vi "EyeTrackerFPGA (FPGA).vi"() -> ()   [LabVIEW 2012]
uses:
  <vilib>/Platform/TimedLoop/XDataNode/timing_clust.ctl
  <vilib>/Platform/TimedLoop/XDataNode/nitl_modes.ctl
  <vilib>/Platform/TimedLoop/XDataNode/wakeup.ctl
  Common/CL Configuration.ctl
  Common/CL Signal Mapping.ctl
  <vilib>/rvi/eio/common/nirviEmuTemplateMethod_errors.vi
  <vilib>/rvi/Emulation/niFpgaSctlEmulationRegisterWithScheduler.vi
  <vilib>/rvi/Emulation/niFpgaSctlEmulationScheduler.vi
  <vilib>/rvi/interface/RandomDataEmulation/nirviRandomDataFPGAFIFO.vi
  <vilib>/rvi/interface/RandomDataEmulation/niFpgaRandomDataHandleErrors.vi
  <vilib>/rvi/DataTransferAndStorage/Container/Common/niFpgaContainerGetUniqueNameForEmu.vi
  <vilib>/rvi/FIFO/Fifo_Resource/nirvififoEmulationSetSize.vi
  <vilib>/rvi/Emulation/niFpgaSctlEmulationFifoFullMgr.vi
  <vilib>/rvi/errors/niFpgaSetErrorForExecOnDevCompSimple.vi
  <vilib>/rvi/eio/common/nirviEmuReportErrorAndStop.vi
  Common/CL Data to Pixels/2 Tap 8-Bit.vi
  Common/CL Data to Pixels/2 Tap 10-Bit.vi
  <vilib>/rvi/Emulation/niFpgaSctlEmulationGlobalWrite.vi
  <vilib>/rvi/Emulation/niFpgaSctlEmulationResourceMgr.vi
  <vilib>/Platform/TimedLoop/XDataNode/XDataNode.xnode
  <vilib>/eio/EIONode/EIONode.xnode
  <vilib>/rvi/FXPMathLib/FxpInterpret/XNode/nifxpmath_Interpret.xnode
  <vilib>/rvi/DataTransferAndStorage/Container/XNode/niFpgaContainer.xnode
  <vilib>/rvi/interface/RandomDataEmulation/nirviRandomDataFpgaReadWriteTemplate.vi
  <vilib>/rvi/FIFO/Fifo_Resource/nirvififoEmulationRead.vi
  <vilib>/rvi/FIFO/Fifo_Resource/nirvififoEmulationWrite.vi
  <vilib>/Platform/TimedLoop/XDataNode/XDNodeRunTimeDep.lvlib
panel:
  in  "10-bit":bool
  out "Fixation.Fixated":bool
  in  "Fixation.MaxY":fxp<+/-,64,33> format="%.41g"
  in  "Fixation.MinY":fxp<+/-,64,33> format="%.41g"
  in  "Fixation.MaxX":fxp<+/-,64,33> format="%.41g"
  in  "Fixation.MinX":fxp<+/-,64,33> format="%.41g"
  in  "Fixation.MinimumEyeSize":u32
  out "AcqStatus.BufferToHostFull":bool
  out "AcqStatus.TenFrameTime":u32
  out "AcqStatus.DataAvailable":u32
  out "AcqStatus.PushedToHost":u32
  out "AcqStatus.PushedToMem":u32
  out "Acq Status.FrameWidth":u32
  out "Acq Status.FrameHeight":u32
  out "Acq Status.FrameNum":u32
  out "Acq Status.Acq'd Frame Width":u32
  out "Acq Status.Frames Acq'd":u32
  out "Acq Status.Acq'd Frame Height":u32
  out "Acq Status.DMA Write Timeout":bool
  out "Acq Status.Initialized":bool
  in  "EyePosition.Shift":i8=-2
  out "Timed Out?":bool
  out "Centroid.NumSent":i32
  out "Centroid.SumY":u32
  out "Centroid.SumX":u32
  out "Centroid.Size":u32
  out "Grabbed":bool
  out "Grabbing":bool
  in  "EyePosition.Color":u8=100
  in  "EyePosition.Send":bool
  in  "EyePosition.Threshold":u16=10
  out "TestX":u32
  out "TestY":u32
  in  "UART.Baud Rate":u8
  in  "UART.Transmit":bool
  in  "UART.Tx Data":u8[](array[numeric])=[0, 0, 0, 0, 0, 0, 0, 0, 0, 0] format="%02x"
  in  "UART.Set Baud Rate":bool
  in  "UART.Byte Mode":bool=TRUE
  out "UART.Rx Ready":bool
  out "UART.Break Indicator":bool
  out "UART.Framing Error":bool
  out "UART.Overrun Error":bool
  out "UART.Tx Ready":bool
  out "UART.Rx Data":u8 format="%02x"
  in  "UART.Receive":bool
  in  "Acq Control.Grab":bool
  in  "Acq Control.Acq":bool
  in  "Acq Control.IgnoreDVAL":bool
  in  "Acq Control.Clear Frame Cnt":bool
  in  "Acq Control.Initialize":bool
  in  "Trigger.Trigger Pulse Width (40 MHz Ticks)":u32=4000
  in  "Trigger.Send Software Trigger":bool
  in  "IO Module Config.CL DVAL Active High":bool=TRUE
  in  "IO Module Config.CL LVAL Active High":bool=TRUE
  in  "IO Module Config.CL FVAL Active High":bool=TRUE
  in  "IO Module Config.CL Spare Active High":bool=TRUE
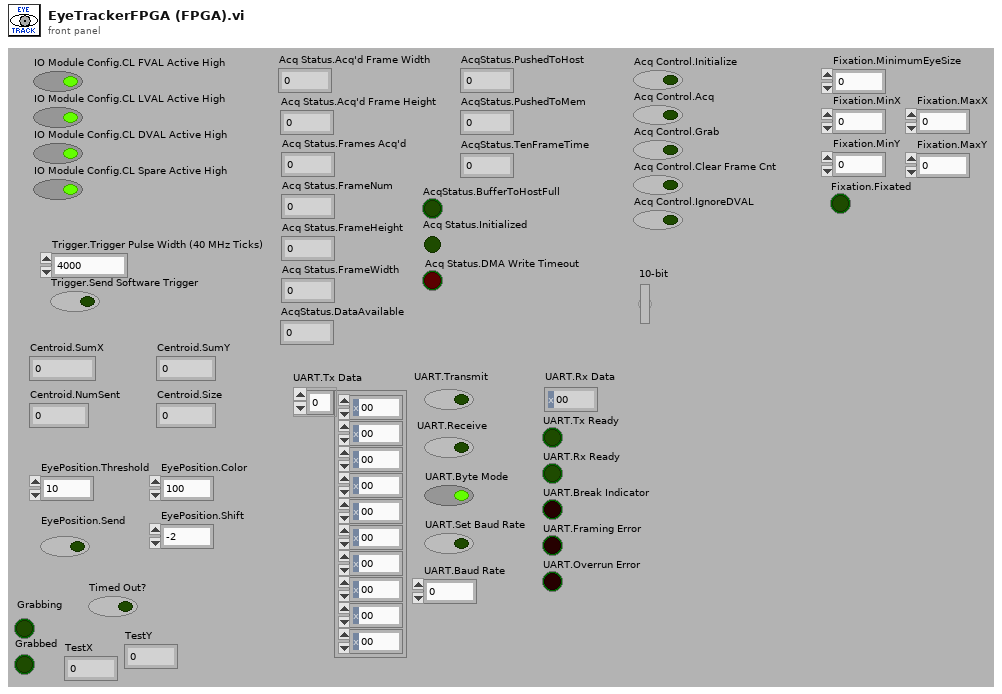
[diagram p1: front panel]
types:
  T1 = typedef "CL Signal Mapping.ctl" = enum8{"Standard", "Basler 10-tap", "Vosskühler 10-tap"}
  T2 = typedef "CL Configuration.ctl" = enum8{"Base", "Medium", "Full"}
  T3 = typedef "XDNodeRunTimeDep.lvlib/timing_clust.ctl" = cluster{"Expected End [f-1]":u64, "Actual End [f-1]":u64, "Finished Late? [f-1]":bool, "Expected End [i-1]":u64, "Actual End [i-1]":u64, "Finished Late? [i-1]":bool, "Expected Start [i]":u64, "Actual Start [i]":u64, "Expected Start [f]":u64, "Actual Start [f]":u64, "Source Name":string, "Structure Name":string, "Period":i64, "Deadline":i64, "Offset":i64, "Start":i64, "Priority":i32, "Timeout":i32, "Mode":T4, "Wakeup Reason":T5, "Error":errorcluster, "Source Type":string, "Secondary Source Type":string, "Global End Time":u64, "Global Start Time":u64, "Frame Duration":u64, "Iteration Duration":u64, "Assigned CPU":i32, "I/O Scan Engine Mode":u32}
  T4 = typedef "XDNodeRunTimeDep.lvlib/nitl_modes.ctl" = enum32{"No Change", "Process missed periods, maintain original phase", "Discard missed periods, maintain original phase", "Process missed periods, ignore original phase", "Discard missed periods, ignore original phase"}
  T5 = typedef "XDNodeRunTimeDep.lvlib/wakeup.ctl" = enum32{"Normal", "Aborted", "Asynchronous wakeup", "Timing source error", "Timed loop error", "Timeout"}
  T6 = enum16{"Idle", "WaitForPreviousEnd", "WaitForFrameRising", "WaitForFrameFalling", "CheckIfArmed"}
  T7 = cluster{"Tx Data":u8[], "Transmit":bool, "Receive":bool, "Byte Mode":bool, "Set Baud Rate":bool, "Baud Rate":u8}
  T8 = cluster{"Rx Data":u8, "Turn Off Transmit":bool, "Turn Off Receive":bool, "Turn Off Set Baud Rate":bool, "Tx Ready":bool, "Rx Ready":bool, "Break Indicator":bool, "Framing Error":bool, "Overrun Error":bool}
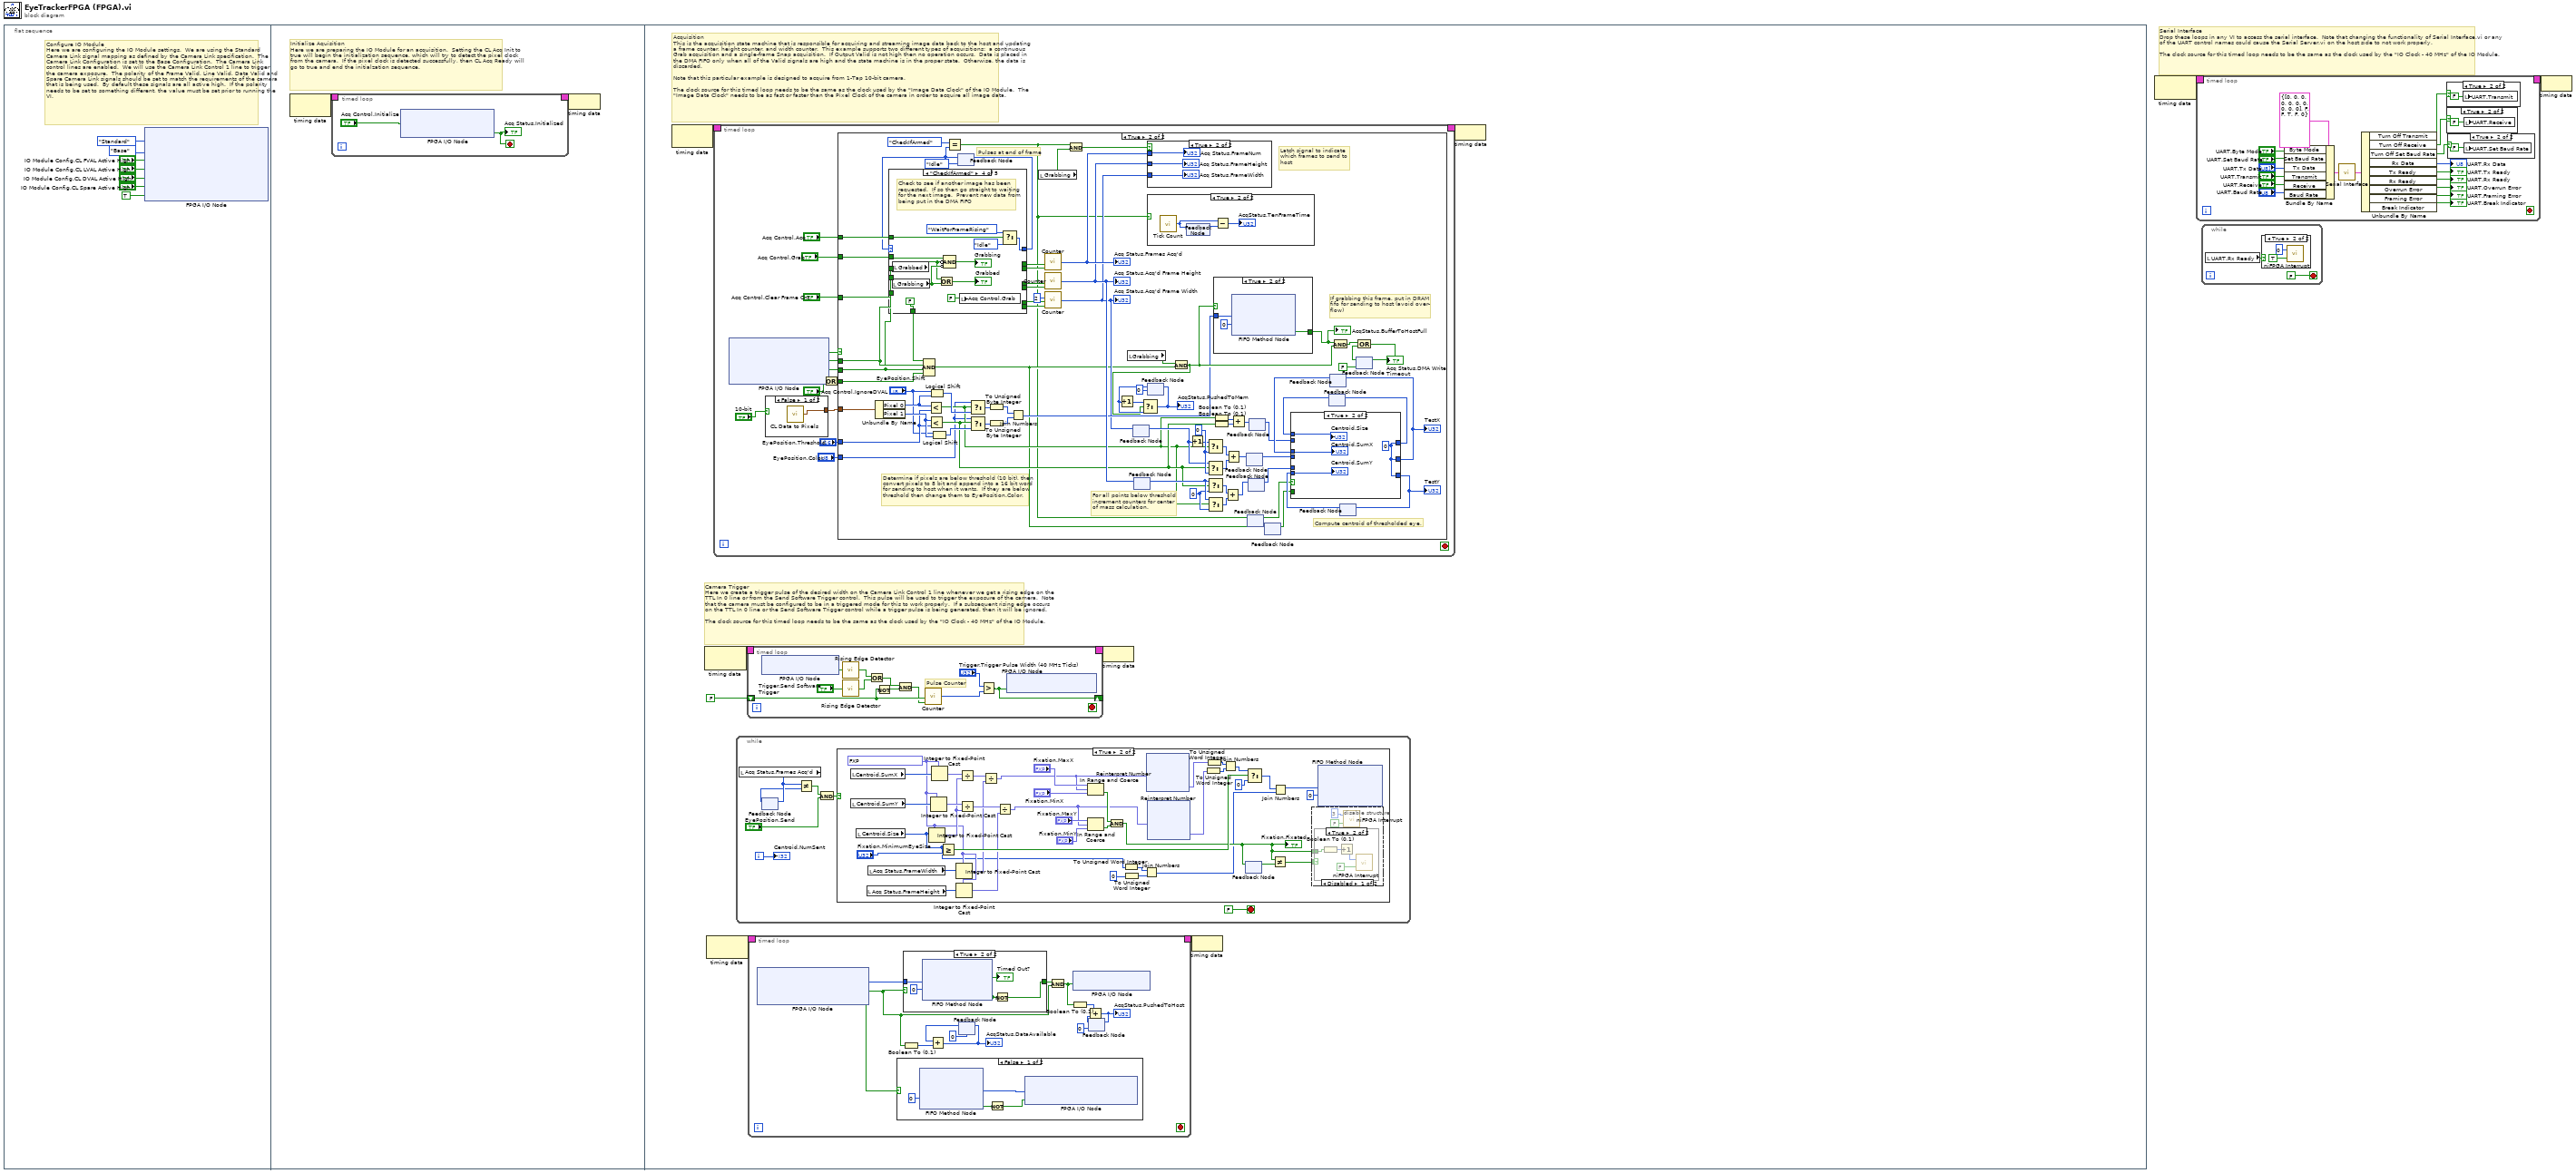
[diagram p0: block diagram]
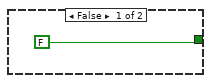
[diagram p7: hidden frame]
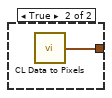
[diagram p11: hidden frame]
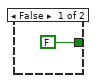
[diagram p14: hidden frame]
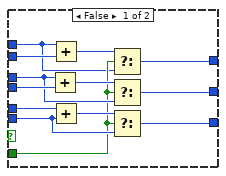
[diagram p16: hidden frame]
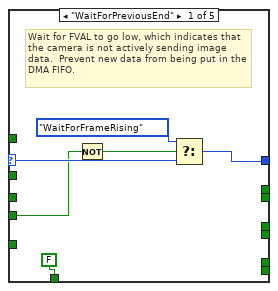
[diagram p17: hidden frame]
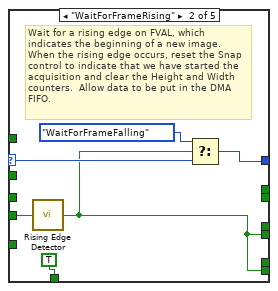
[diagram p18: hidden frame]
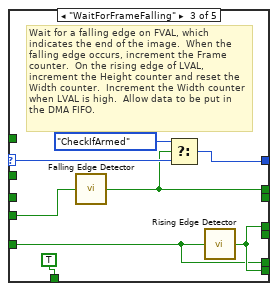
[diagram p19: hidden frame]
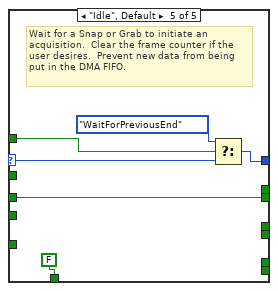
[diagram p20: hidden frame]
diagram:
  # "Serial Interface\nDrop these loops in any VI to access the serial interface.  Note that changing the functionality of Serial Interface.vi or any of the UART control names could cause the Serial Server.vi on the host side to not work properly.\n\nThe clock source for this timed loop needs to be the same as the clock used by the \"IO Clock - 40 MHz\" of the IO Module."
  n1 = flat-sequence {
    frame #0 {
      # "Configure IO Module\nHere we are configuring the IO Module settings.  We are using the Standard Camera Link signal mapping as defined by the Camera Link specification.  The Camera Link Configuration is set to the Base Configuration.  The Camera Link control lines are enabled.  We will use the Camera Link Control 1 line to trigger the camera exposure.  The polarity of the Frame Valid, Line Valid, Data Valid and Spare Camera Link signals should be set to match the requirements of the camera that is being used.  By default these signals are all active high.  If the polarity needs to be set to something different, the value must be set prior to running the VI."
      n2 = xnode "FPGA I/O Node"("IO Module\\CL Set Signal Mapping"=CL_Signal_Mapping."Standard" ("Camera Link Data Mapping"), "IO Module\\CL Set Configuration"=CL_Configuration."Base" ("CL Configuration"), "IO Module\\CL Set FVAL Active High"="IO Module Config.CL FVAL Active High", "IO Module\\CL Set LVAL Active High"="IO Module Config.CL LVAL Active High", "IO Module\\CL Set DVAL Active High"="IO Module Config.CL DVAL Active High", "IO Module\\CL Set Spare Active High"="IO Module Config.CL Spare Active High", "IO Module\\CL Control Enable"=TRUE ("IO Module\\CL Set Spare Active High")) -> ()  [unwired: 7 in, 7 out]
    }
    frame #1 {
      # "Initialize Aquisition\nHere we are preparing the IO Module for an acquisition.  Setting the CL Acq Init to true will begin the initialization sequence, which will try to detect the pixel clock from the camera.  If the pixel clock is detected successfully, then CL Acq Ready will go to true and end the initialzation sequence."
      n3 = node-c288() -> (w11:T3)  [unwired: 1 out]
      n4 = timed-loop {
        timing: w11 -> [_]
        timing-out: [_] -> w10
        stop <- w12 stop-if-true
        n5 = xnode "FPGA I/O Node"("IO Module\\CL Acq Init"="Acq Control.Initialize") -> ("IO Module\\CL Acq Ready"=w12:bool)  [unwired: 2 in, 2 out]
        "Acq Status.Initialized" <- w12
      }
      n6 = node-c288(w10) -> ()
    }
    frame #2 {
      # "Acquisition\nThis is the acquisition state machine that is responsible for acquiring and streaming image data back to the host and updating a frame counter, height counter, and width counter.  This example supports two different types of acquisitions:  a continuous Grab acquisition and a single-frame Snap acquisition.  If Output Valid is not high then no operation occurs.  Data is placed in the DMA FIFO only when all of the Valid signals are high and the state machine is in the proper state.  Otherwise, the data is discarded.\n\nNote that this particular example is designed to acquire from 1-Tap 10-bit camera.\n\nThe clock source for this timed loop needs to be the same as the clock used by the \"Image Data Clock\" of the IO Module.  The \"Image Data Clock\" needs to be as fast or faster than the Pixel Clock of the camera in order to acquire all image data."
      # "Camera Trigger\nHere we create a trigger pulse of the desired width on the Camera Link Control 1 line whenever we get a rising edge on the TTL In 0 line or from the Send Software Trigger control.  This pulse will be used to trigger the exposure of the camera.  Note that the camera must be configured to be in a triggered mode for this to work properly.  If a subsequent rising edge occurs on the TTL In 0 line or the Send Software Trigger control while a trigger pulse is being generated, then it will be ignored. \n\nThe clock source for this timed loop needs to be the same as the clock used by the \"IO Clock - 40 MHz\" of the IO Module."
      n7 = node-c288() -> (w24:T3)  [unwired: 1 in]
      n8 = node-c288() -> (w22:T3)  [unwired: 1 in]
      n9 = node-c288() -> (w19:T3)  [unwired: 1 in]
      n10 = timed-loop {
        timing: w24 -> [_]
        timing-out: [_] -> w23
        stop <- _ stop-if-true
        n11 = xnode "FPGA I/O Node"() -> ("IO Module\\CL Output Valid"=w132:bool, "IO Module\\CL Frame Valid"=w131:bool, "IO Module\\CL Line Valid"=w130:bool, "IO Module\\CL Data Valid"=w128:bool)  [unwired: 4 in, 4 out]
        n12 = case shown="False" "10-bit" {
          tunnel: [w133 w134] -> w126
          frame False {
            n13 = call-poly "CL Data to Pixels.vi"() -> ("PixelData"=w133:cluster{"Pixel 0":u8, "Pixel 1":u8})  [unwired: 1 in]
          }
          frame True {
            n14 = call-poly "CL Data to Pixels.vi"() -> ("PixelData"=w134:cluster{"Pixel 0":u16, "Pixel 1":u16})  [unwired: 1 in]
          }
        }
        n15 = Or(x=w128, y="Acq Control.IgnoreDVAL") -> (x .or. y?=w127:bool)
        n16 = case shown="True" w132 {
          tunnel: w131 -> [_ w206]
          tunnel: w130 -> [_ w196]
          tunnel: w127 -> [_ w205]
          tunnel: w126 -> [_ w194]
          tunnel: "Acq Control.Acq" -> [_ w204]
          tunnel: "Acq Control.Clear Frame Cnt" -> [_ w203]
          tunnel: "EyePosition.Threshold" -> [_ w177]
          tunnel: "Acq Control.Grab" -> [_ w166]
          tunnel: "EyePosition.Color" -> [_ w145]
          frame False {
          }
          frame True {
            w174 = i16 0
            w193 = u32 0
            # "If grabbing this frame, put in DRAM\nfifo for sending to host (avoid over-\nflow)"
            # "For all points below threshold\nincrement counters for center\nof mass calculation."
            # "Determine if pixels are below threshold (10 bit), then\nconvert pixels to 8 bit and append into a 16 bit word\nfor sending to host when it wants.  If they are below \nthreshold then change them to EyePosition.Color."
            # "Pulses at end of frame"
            # "Latch signal to indicate \nwhich frames to send to \nhost"
            # "Compute centroid of thresholded eye,"
            n17 = Unbundle By Name(w194) -> ("Pixel 0"=w179:u16, "Pixel 1"=w178:u16)
            n18 = Less?(x=w179, y=w177) -> (x < y?=w163:bool)
            n19 = Less?(x=w178, y=w177) -> (x < y?=w164:bool)
            n20 = Logical Shift(y="EyePosition.Shift", x=w179) -> (x << y=w181:u16)
            n21 = Logical Shift(y="EyePosition.Shift", x=w178) -> (x << y=w180:u16)
            n22 = feedback #1(T6."Idle") -> (w167:T6)
            n23 = case shown="\"CheckIfArmed\"" w167 {
              selector: w167 -> [w240 w248 w256 _ w273]
              tunnel: [w241 w249 w257 w267 w274] -> w170
              tunnel: [FALSE TRUE TRUE FALSE FALSE] -> w208
              tunnel: w204 -> [_ _ _ w265 w270]
              tunnel: w206 -> [w239 w246 w253 _ _]
              tunnel: w203 -> [_ _ _ _ w269]
              tunnel: [_ _ w252 _ _] -> w202
              tunnel: [_ _ _ _ w269] -> w201
              tunnel: [_ _ w251 _ _] -> w200
              tunnel: [_ w244 _ _ _] -> w199
              tunnel: [_ _ w250 _ _] -> w198
              tunnel: [_ w244 w251 _ _] -> w197
              tunnel: w196 -> [_ _ w250 _ _]
              tunnel: w166 -> [_ _ _ w262 _]
              frame "WaitForPreviousEnd" {
                # "Wait for FVAL to go low, which indicates that the camera is not actively sending image data.  Prevent new data from being put in the DMA FIFO."
                n24 = Not(x=w239) -> (.not. x?=w238:bool)
                n25 = Select(t=T6."WaitForFrameRising", s=w238, f=w240) -> (s? t:f=w241:T6)
              }
              frame "WaitForFrameRising" {
                # "Wait for a rising edge on FVAL, which indicates the beginning of a new image.  When the rising edge occurs, reset the Snap control to indicate that we have started the acquisition and clear the Height and Width counters.  Allow data to be put in the DMA FIFO."
                n26 = call "Rising Edge Detector.vi"("Signal In"=w246) -> ("Edge Detected?"=w244:bool)
                n27 = Select(t=T6."WaitForFrameFalling", s=w244, f=w248) -> (s? t:f=w249:T6)
              }
              frame "WaitForFrameFalling" {
                # "Wait for a falling edge on FVAL, which indicates the end of the image.  When the falling edge occurs, increment the Frame counter.  On the rising edge of LVAL, increment the Height counter and reset the Width counter.  Increment the Width counter when LVAL is high.  Allow data to be put in the DMA FIFO."
                n28 = call "Falling Edge Detector.vi"("Signal In"=w253) -> ("Edge Detected?"=w252:bool)
                n29 = Select(t=T6."CheckIfArmed", s=w252, f=w256) -> (s? t:f=w257:T6)
                n30 = call "Rising Edge Detector.vi"("Signal In"=w250) -> ("Edge Detected?"=w251:bool)
              }
              frame "CheckIfArmed" {
                # "Check to see if another image has been requested.  If so then go straight to waiting for the next image.  Prevent new data from being put in the DMA FIFO"
                n31 = local read "Grabbing"() -> (w260:bool)
                n32 = local read "Grabbed"() -> (w258:bool)
                n33 = Or(x=w258, y=w260) -> (x .or. y?=→"Grabbed":bool)
                n34 = Compound Arithmetic op=AND(w262, invert w258, invert w260) -> (→"Grabbing":bool)
                n35 = local write "Acq Control.Grab"(FALSE ("Acq Control.Grab")) -> ()
                n36 = Select(t=T6."WaitForFrameRising", s=w265, f=T6."Idle") -> (s? t:f=w267:T6)
              }
              frame "Idle", Default {
                # "Wait for a Snap or Grab to initiate an acquisition.  Clear the frame counter if the user desires.  Prevent new data from being put in the DMA FIFO."
                n37 = Select(t=T6."WaitForPreviousEnd", s=w270, f=w273) -> (s? t:f=w274:T6)
              }
            }
            n38 = Compound Arithmetic op=AND(w208, w206, w196, w205) -> (w144:bool)
            n39 = Equal?(x=T6."CheckIfArmed" ("y"), y=w167) -> (x = y?=w142:bool)
            n40 = feedback-in #1(w170) -> ()
            n41 = Select(t=w145, s=w163, f=w181) -> (s? t:f=w182:u16)
            n42 = Select(t=w145, s=w164, f=w180) -> (s? t:f=w183:u16)
            n43 = To Unsigned Byte Integer(number=w182) -> (unsigned 8bit integer=w184:u8)
            n44 = To Unsigned Byte Integer(number=w183) -> (unsigned 8bit integer=w185:u8)
            n45 = Join Numbers(hi=w184, lo=w185) -> ((hi.lo)=w150:u16)
            n46 = local read "Grabbing"() -> (w158:bool)
            n47 = call "Counter.vi"("Reset?"=w201, "Increment?"=w202) -> ("Value"=w169:u32)  [unwired: 2 in]
            "Acq Status.Frames Acq'd" <- w169
            n48 = call "Counter.vi"("Reset?"=w199, "Increment?"=w200) -> ("Value"=w168:u32)  [unwired: 2 in]
            "Acq Status.Acq'd Frame Height" <- w168
            n49 = call "Counter.vi"("Reset?"=w197, "Increment?"=w198, "Increment Value"=u32 2) -> ("Value"=w147:u32)  [unwired: 1 in]
            "Acq Status.Acq'd Frame Width" <- w147
            n50 = And(x=w142, y=w158) -> (x .and. y?=w157:bool)
            n51 = local read "Grabbing"() -> (w165:bool)
            n52 = feedback-in #2(w147) -> ()
            n53 = feedback #2() -> (w176:u32)  [unwired: 1 in]
            n54 = feedback-in #3(w168) -> ()
            n55 = feedback #3() -> (w175:u32)  [unwired: 1 in]
            n56 = case shown="True" w142 {
              frame False {
              }
              frame True {
                n57 = call "Tick Count"() -> ("Tick Count(uSec)"=w213:u32)
                n58 = feedback-in #4(w213) -> ()
                n59 = feedback #4() -> (w212:u32)  [unwired: 1 in]
                n60 = Subtract(x=w213, y=w212) -> (x-y=→"AcqStatus.TenFrameTime":u32)
              }
            }
            n61 = feedback #5(u32 0) -> (w152:u32)
            n62 = Increment(x=w152) -> (x+1=w154:u32)
            n63 = case shown="True" w157 {
              tunnel: w169 -> [_ w220]
              tunnel: w168 -> [_ w219]
              tunnel: w147 -> [_ w218]
              frame False {
              }
              frame True {
                "Acq Status.FrameNum" <- w220
                "Acq Status.FrameHeight" <- w219
                "Acq Status.FrameWidth" <- w218
              }
            }
            n64 = And(x=w165, y=w144) -> (x .and. y?=w151:bool)
            n65 = Select(t=w154, s=w151, f=w152) -> (s? t:f=w153:u32)
            "AcqStatus.PushedToMem" <- w153
            n66 = feedback-in #5(w153) -> ()
            n67 = Increment(x=w176) -> (x+1=w192:u32)
            n68 = Select(t=w192, s=w163, f=w193) -> (s? t:f=w191:u32)
            n69 = Select(t=w176, s=w164, f=w193) -> (s? t:f=w190:u32)
            n70 = Select(t=w175, s=w164, f=w174) -> (s? t:f=w173:u32)
            n71 = Select(t=w175, s=w163, f=w174) -> (s? t:f=w172:u32)
            n72 = case shown="True" w151 {
              tunnel: w150 -> [_ w217]
              tunnel: [FALSE ("Timed Out?") w215] -> w149
              frame False {
              }
              frame True {
                n73 = xnode ("FIFO Method Node")("Element"=w217, "Timeout"=0) -> ("Timed Out?"=w215:bool)  [unwired: 1 in, 1 out]
              }
            }
            "AcqStatus.BufferToHostFull" <- w149
            n74 = Boolean To (0,1)(Boolean=w163) -> (0, 1=w161:i16)
            n75 = Boolean To (0,1)(Boolean=w164) -> (0, 1=w162:i16)
            n76 = Add(x=w173, y=w172) -> (x+y=w140:u32)
            n77 = Add(x=w191, y=w190) -> (x+y=w138:u32)
            n78 = Add(x=w161, y=w162) -> (x+y=w136:i16)
            n79 = feedback-in #6(w138) -> ()
            n80 = feedback #6() -> (w137:u32)  [unwired: 1 in]
            n81 = feedback-in #7(w142) -> ()
            n82 = feedback #7() -> (w141:bool)  [unwired: 1 in]
            n83 = feedback-in #8(w140) -> ()
            n84 = feedback #8() -> (w139:u32)  [unwired: 1 in]
            n85 = feedback-in #9(w136) -> ()
            n86 = feedback #9() -> (w135:i16)  [unwired: 1 in]
            n87 = feedback-in #10(w144) -> ()
            n88 = feedback #10() -> (w143:bool)  [unwired: 1 in]
            n89 = feedback #11() -> (w159:u32)  [unwired: 1 in]
            n90 = feedback #12() -> (w188:u32)  [unwired: 1 in]
            n91 = And(x=w149, y=w151) -> (x .and. y?=w156:bool)
            n92 = feedback #13() -> (w186:u32)  [unwired: 1 in]
            n93 = case shown="True" w141 {
              tunnel: w137 -> [w233 _]
              tunnel: [w222 w237] -> w189
              tunnel: w188 -> [w227 w235]
              tunnel: [w221 w237] -> w187
              tunnel: w186 -> [w229 w234]
              tunnel: w139 -> [w232 _]
              tunnel: w143 -> [w226 _]
              tunnel: w159 -> [w224 w236]
              tunnel: [w223 w237] -> w160
              tunnel: w135 -> [w231 _]
              frame False {
                n94 = Add(x=w227, y=w233) -> (x+y=w228:u32)
                n95 = Add(x=w224, y=w231) -> (x+y=w225:u32)
                n96 = Add(x=w232, y=w229) -> (x+y=w230:u32)
                n97 = Select(t=w225, s=w226, f=w224) -> (s? t:f=w223:u32)
                n98 = Select(t=w228, s=w226, f=w227) -> (s? t:f=w222:u32)
                n99 = Select(t=w230, s=w226, f=w229) -> (s? t:f=w221:u32)
              }
              frame True {
                w237 = u32 0
                "Centroid.Size" <- w236
                "Centroid.SumX" <- w235
                "Centroid.SumY" <- w234
              }
            }
            "TestY" <- w187
            "TestX" <- w189
            n100 = feedback-in #11(w160) -> ()
            n101 = feedback-in #12(w189) -> ()
            n102 = feedback-in #13(w187) -> ()
            n103 = feedback #14(FALSE) -> (w209:bool)
            n104 = Compound Arithmetic op=OR(w156, w209) -> (w207:bool)
            "Acq Status.DMA Write Timeout" <- w207
            n105 = feedback-in #14(w207) -> ()
          }
        }
      }
      n106 = while {
        i -> [w51]
        stop <- FALSE stop-if-true
        n107 = local read "Acq Status.Frames Acq'd"() -> (w56:u32)
        n108 = feedback-in #15(w56) -> ()
        n109 = feedback #15() -> (w55:u32)  [unwired: 1 in]
        n110 = Not Equal?(x=w56, y=w55) -> (x != y?=w54:bool)
        n111 = And(x=w54, y="EyePosition.Send") -> (x .and. y?=w52:bool)
        n112 = case shown="True" w52 {
          frame False {
          }
          frame True {
            w71 = fxp<+/-,32,32> 0.0 ("fixed-point type")
            n113 = local read "Centroid.SumX"() -> (w96:u32)
            n114 = local read "Centroid.SumY"() -> (w94:u32)
            n115 = local read "Centroid.Size"() -> (w64:u32)
            n116 = local read "Acq Status.FrameHeight"() -> (w72:u32)
            n117 = local read "Acq Status.FrameWidth"() -> (w73:u32)
            n118 = Integer to Fixed-Point Cast(fixed-point type=w71, integer=w64) -> (fixed-point=w90:fxp<+/-,32,32>)
            n119 = Integer to Fixed-Point Cast(fixed-point type=w71, integer=w94) -> (fixed-point=w93:fxp<+/-,32,32>)
            n120 = Integer to Fixed-Point Cast(fixed-point type=w71, integer=w96) -> (fixed-point=w95:fxp<+/-,32,32>)
            n121 = Greater Or Equal?(x=w64, y="Fixation.MinimumEyeSize") -> (x >= y?=w86:bool)
            n122 = Integer to Fixed-Point Cast(fixed-point type=w71, integer=w73) -> (fixed-point=w68:fxp<+/-,32,32>)
            n123 = Integer to Fixed-Point Cast(fixed-point type=w71, integer=w72) -> (fixed-point=w67:fxp<+/-,32,32>)
            n124 = Divide(x=w95, y=w90) -> (x/y=w70:fxp<+/-,64,33>)
            n125 = Divide(x=w93, y=w90) -> (x/y=w69:fxp<+/-,64,33>)
            n126 = Divide(x=w70, y=w68) -> (x/y=w66:fxp<+/-,64,34>)
            n127 = Divide(x=w69, y=w67) -> (x/y=w65:fxp<+/-,64,34>)
            n128 = In Range and Coerce(upper limit="Fixation.MaxX", x=w66, lower limit="Fixation.MinX") -> (In Range?=w77:bool)  [unwired: 1 out]
            n129 = In Range and Coerce(upper limit="Fixation.MaxY", x=w65, lower limit="Fixation.MinY") -> (In Range?=w78:bool)  [unwired: 1 out]
            n130 = And(x=w77, y=w78) -> (x .and. y?=w74:bool)
            "Fixation.Fixated" <- w74
            n131 = To Unsigned Word Integer(number=w64) -> (unsigned 16bit integer=w62:u16)
            n132 = To Unsigned Word Integer(number=u16 0) -> (unsigned 16bit integer=w61:u16)
            n133 = Join Numbers(hi=w62, lo=w61) -> ((hi.lo)=w59:u32)
            n134 = xnode "Reinterpret Number"("x"=w66) -> ("y"=w83:fxp<+,64,49>)
            n135 = xnode "Reinterpret Number"("x"=w65) -> ("y"=w88:fxp<+,64,49>)
            n136 = To Unsigned Word Integer(number=w88) -> (unsigned 16bit integer=w91:u16)
            n137 = To Unsigned Word Integer(number=w83) -> (unsigned 16bit integer=w92:u16)
            n138 = Join Numbers(hi=w92, lo=w91) -> ((hi.lo)=w85:u32)
            n139 = feedback-in #16(w74) -> ()
            n140 = feedback #16() -> (w76:bool)  [unwired: 1 in]
            n141 = Select(t=w85, s=w86, f=u32 0) -> (s? t:f=w60:u32)
            n142 = Not Equal?(x=w74, y=w76) -> (x != y?=w75:bool)
            n143 = Join Numbers(hi=w60, lo=w59) -> ((hi.lo)=w58:u64)
            n144 = disable-structure shown="Disabled" {
              disable-tunnel: w75 -> [w98 _]
              disable-tunnel: w74 -> [w97 _]
              frame Disabled {
                n145 = case shown="True" w98 {
                  tunnel: w97 -> [_ w103]
                  frame False {
                  }
                  frame True {
                    n146 = Boolean To (0,1)(Boolean=w103) -> (0, 1=w102:i16)
                    n147 = Increment(x=w102) -> (x+1=w101:i16)
                    n148 = call <vilib>:"niFPGA Interrupt.vi"("Wait Until Cleared (F)"=FALSE ("Wait Until Cleared"), "IRQ Number (0)"=w101) -> ()  [unwired: 1 in]
                  }
                }
                n149 = call <vilib>:"niFPGA Interrupt.vi"("Wait Until Cleared (F)"=FALSE ("Wait Until Cleared"), "IRQ Number (0)"=u8 3 ("IRQ Number")) -> ()  [unwired: 1 in]
              }
              frame Enabled {
              }
            }
            n150 = xnode ("FIFO Method Node")("Element"=w58, "Timeout"=0) -> ()  [unwired: 1 in, 2 out]
          }
        }
        "Centroid.NumSent" <- w51
      }
      n151 = timed-loop {
        timing: w22 -> [_]
        timing-out: [_] -> w21
        shift-right: [w109] -> _
        shift-left: FALSE -> [w106]
        stop <- _ stop-if-true
        # "Pulse Counter"
        n152 = xnode "FPGA I/O Node"() -> ("IO Module\\TTL In 0"=w113:bool)  [unwired: 1 in, 1 out]
        n153 = call "Rising Edge Detector.vi"("Signal In"=w113) -> ("Edge Detected?"=w112:bool)
        n154 = call "Rising Edge Detector.vi"("Signal In"="Trigger.Send Software Trigger") -> ("Edge Detected?"=w114:bool)
        n155 = Or(x=w112, y=w114) -> (x .or. y?=w108:bool)
        n156 = Not(x=w106) -> (.not. x?=w107:bool)
        n157 = And(x=w108, y=w107) -> (x .and. y?=w105:bool)
        n158 = call "Counter.vi"("Reset?"=w105, "Increment?"=w106) -> ("Value"=w110:u32)  [unwired: 2 in]
        n159 = Greater?(x="Trigger.Trigger Pulse Width (40 MHz Ticks)", y=w110) -> (0:w109:bool)
        n160 = xnode "FPGA I/O Node"("IO Module\\CL Control 1"=w109) -> ()  [unwired: 1 in, 1 out]
      }
      n161 = timed-loop {
        timing: w19 -> [_]
        timing-out: [_] -> w18
        stop <- _ stop-if-true
        n162 = xnode "FPGA I/O Node"() -> ("BufferToHost\\Read_Data_Upper"=w37:u32, "BufferToHost\\Data_Available"=w25:bool, "BufferToHost\\Full"=w27:bool)  [unwired: 3 in, 3 out]
        n163 = case shown="False" w27 {
          frame False {
            n164 = xnode ("FIFO Method Node")("Timeout"=0) -> ("Element"=w41:u16, "Timed Out?"=w39:bool)  [unwired: 1 in, 1 out]
            n165 = Not(x=w39) -> (.not. x?=w38:bool)
            n166 = xnode "FPGA I/O Node"("BufferToHost\\Write_Data_Upper"=w41, "BufferToHost\\Write"=w38) -> ()  [unwired: 2 in, 2 out]
          }
          frame True {
          }
        }
        n167 = case shown="True" w25 {
          tunnel: w37 -> [_ w45]
          tunnel: [FALSE ("BufferToHost\\Read") w43] -> w26
          frame False {
          }
          frame True {
            n168 = xnode ("FIFO Method Node")("Element"=w45, "Timeout"=0) -> ("Timed Out?"=w44:bool)  [unwired: 1 in, 1 out]
            "Timed Out?" <- w44
            n169 = Not(x=w44) -> (.not. x?=w43:bool)
          }
        }
        n170 = Boolean To (0,1)(Boolean=w25) -> (0, 1=w34:i16)
        n171 = feedback #17(u32 0) -> (w33:u32)
        n172 = Add(x=w33, y=w34) -> (x+y=w36:u32)
        "AcqStatus.DataAvailable" <- w36
        n173 = feedback-in #17(w36) -> ()
        n174 = And(x=w26, y=w25) -> (x .and. y?=w28:bool)
        n175 = Boolean To (0,1)(Boolean=w28) -> (0, 1=w29:i16)
        n176 = xnode "FPGA I/O Node"("BufferToHost\\Read"=w28) -> ()  [unwired: 1 in, 1 out]
        n177 = feedback #18(i16 0) -> (w30:i16)
        n178 = Add(x=w29, y=w30) -> (x+y=w32:i16)
        "AcqStatus.PushedToHost" <- w32
        n179 = feedback-in #18(w32) -> ()
      }
      n180 = node-c288(w21) -> ()
      n181 = node-c288(w18) -> ()
      n182 = node-c288(w23) -> ()
    }
  }
  n183 = node-c288() -> (w2:T3)  [unwired: 1 out]
  n184 = timed-loop {
    timing: w2 -> [_]
    timing-out: [_] -> w1
    stop <- _ stop-if-true
    n185 = Bundle By Name(cluster=T7 {"Tx Data"=[0, 0, 0, 0, 0, 0, 0, 0, 0, 0], "Transmit"=FALSE, "Receive"=FALSE, "Byte Mode"=TRUE, "Set Baud Rate"=FALSE, "Baud Rate"=0} ("UART Inputs"), "Byte Mode"="UART.Byte Mode", "Set Baud Rate"="UART.Set Baud Rate", "Tx Data"="UART.Tx Data", "Transmit"="UART.Transmit", "Receive"="UART.Receive", "Baud Rate"="UART.Baud Rate") -> (w279:T7)
    n186 = call "Serial Interface.vi"("UART Inputs"=w279) -> ("UART Outputs"=w291:T8)
    n187 = Unbundle By Name(w291) -> ("Turn Off Transmit"=w284:bool, "Turn Off Receive"=w285:bool, "Turn Off Set Baud Rate"=w281:bool, "Rx Data"=→"UART.Rx Data":u8, "Tx Ready"=→"UART.Tx Ready":bool, "Rx Ready"=→"UART.Rx Ready":bool, "Overrun Error"=→"UART.Overrun Error":bool, "Framing Error"=→"UART.Framing Error":bool, "Break Indicator"=→"UART.Break Indicator":bool)
    n188 = case shown="True" w284 {
      frame False {
      }
      frame True {
        n189 = local write "UART.Transmit"(FALSE ("UART.Transmit")) -> ()
      }
    }
    n190 = case shown="True" w285 {
      frame False {
      }
      frame True {
        n191 = local write "UART.Receive"(FALSE ("UART.Receive")) -> ()
      }
    }
    n192 = case shown="True" w281 {
      frame False {
      }
      frame True {
        n193 = local write "UART.Set Baud Rate"(FALSE ("UART.Receive")) -> ()
      }
    }
  }
  n194 = while {
    stop <- FALSE stop-if-true
    n195 = local read "UART.Rx Ready"() -> (w303:bool)
    n196 = case shown="True" w303 {
      frame False {
      }
      frame True {
        n197 = call <vilib>:"niFPGA Interrupt.vi"("Wait Until Cleared (F)"=TRUE ("Wait Until Cleared"), "IRQ Number (0)"=u8 0 ("IRQ Number")) -> ()  [unwired: 1 in]
      }
    }
  }
  n198 = node-c288(w1) -> ()
